vi "Test Lockin API - SM Sequencer.vi"() -> ()   [LabVIEW 2019]
uses:
  src/Instrument.Lockin/Instrument.Lockin.lvclass
  <vilib>/addons/_JKI Toolkits/Caraya/classes/Test Suite/Test Suite.lvclass
  src/Instrument.DAQ/Typedefs/Get State-enum.ctl
  <vilib>/addons/_JKI Toolkits/Caraya/classes/Assert/Assert Not Error.vi
  <vilib>/addons/_JKI Toolkits/Caraya/classes/Assert/Assert Equal Value_Variant.vi
  <vilib>/addons/_JKI Toolkits/Caraya/classes/Test Suite/Define Test Suite (Default).vi
  src/Instrument.DAQ/Typedefs/DAQ.Config.AO.Range--enum.ctl
  src/Instrument.DAQ/Instrument.DAQ.lvclass
  src/Instrument.DAQ/Typedefs/DAQ.Config.AI.Range--enum.ctl
  src/Instrument.DAQ/Typedefs/DAQ.Config.AI.Coupling--enum.ctl
  src/Instrument.DAQ/Typedefs/DAQ.Configuration--Cluster.ctl
  src/Instrument.DAQ/Typedefs/DAQ.Configuration--Cluster--Array.ctl
  <vilib>/addons/_JKI Toolkits/Caraya/classes/Assert/Assert.lvclass
panel:
  out "Current State":string
  in  "Tests":string
  in  "OK":bool
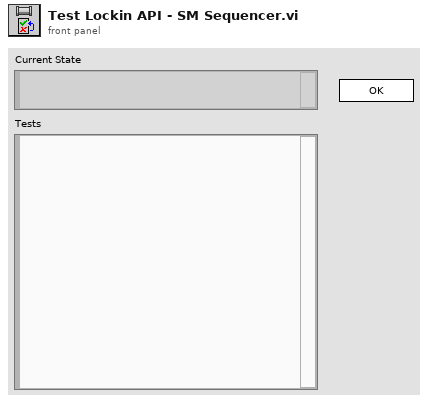
[diagram p1: front panel]
types:
  T1 = typedef "Instrument.DAQ.lvclass/DAQ.Configuration--Cluster--Array.ctl" = T2[]
  T2 = typedef "Instrument.DAQ.lvclass/DAQ.Configuration--Cluster.ctl" = cluster{"Device":string, "AO.Ch":string, "AO.Range":T3, "AI.Ch":string, "AI.Range":T4, "AI.Coupling":T5}
  T3 = typedef "Instrument.DAQ.lvclass/DAQ.Config.AO.Range--enum.ctl" = enum16{"±0.1", "±1.0", "±10.0"}
  T4 = typedef "Instrument.DAQ.lvclass/DAQ.Config.AI.Range--enum.ctl" = enum16{"±0.316", "±1.00", "±3.16", "±10.0", "±31.6", "±42.4"}
  T5 = typedef "Instrument.DAQ.lvclass/DAQ.Config.AI.Coupling--enum.ctl" = u16
  T6 = enum32{"Invalid", "Standard", "Closed", "Hidden", "Minimized", "Maximized"}
  T7 = enum32{"invalid app kind", "Development System", "Run Time System", "Student Edition", "Embedded LabVIEW", "Evaluation", "Custom"}
  T8 = typedef "Instrument.DAQ.lvclass/Get State-enum.ctl" = enum16{"idle", "created", "started", "stopped", "sweeping"}
  T9 = cluster{"Core":cluster{"Current VI Reference":refnum<vi>, "Close Panel on Exit?":bool}, "SelfRef":refnum<class "Instrument.Lockin.lvclass">, "Test Suite":refnum<class "Test Suite.lvclass">}
  T10 = cluster{"Current VI Reference":refnum<vi>, "Close Panel on Exit?":bool}
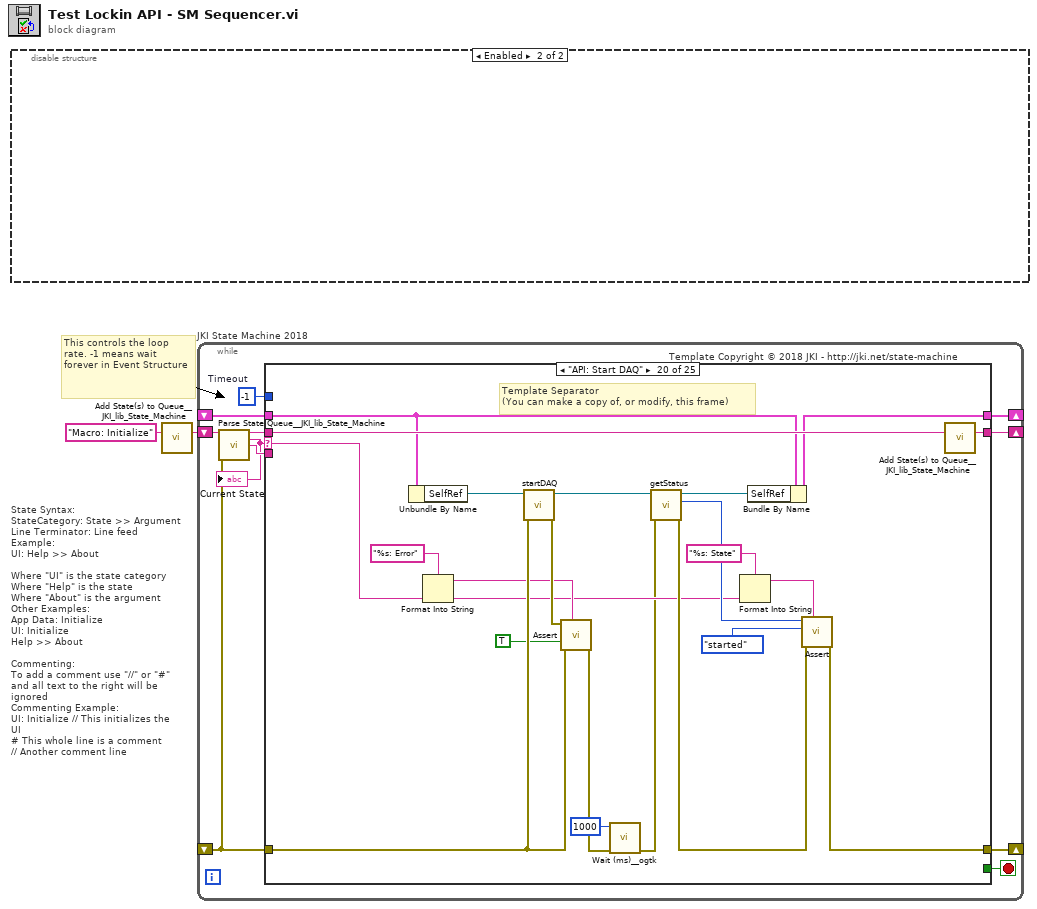
[diagram p0: block diagram]
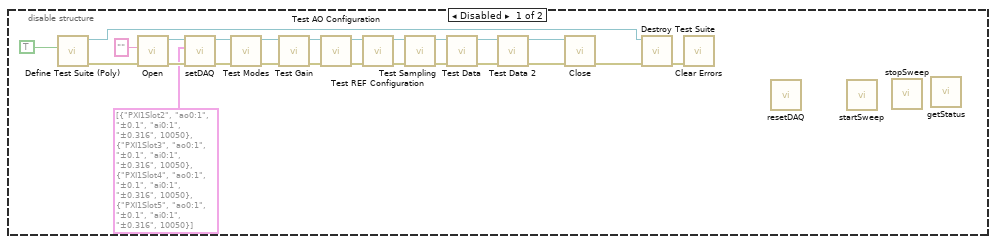
[diagram p2: hidden frame]
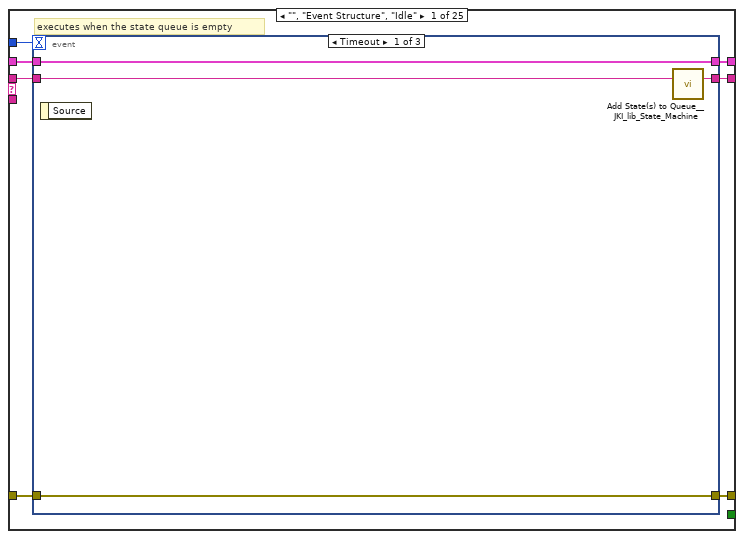
[diagram p3: hidden frame]
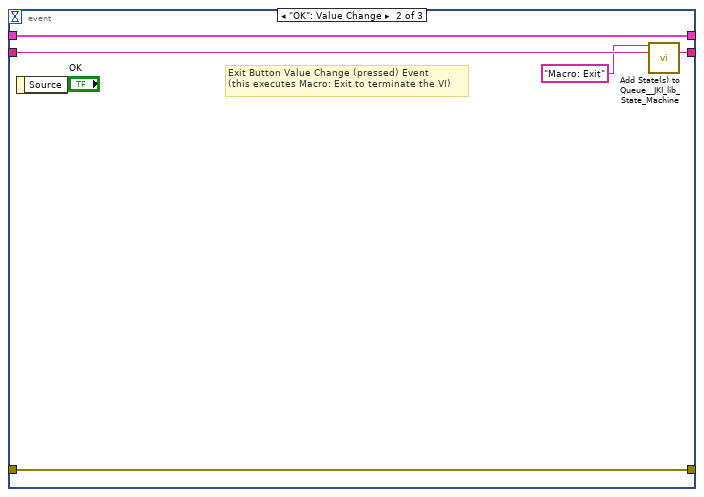
[diagram p4: hidden frame]
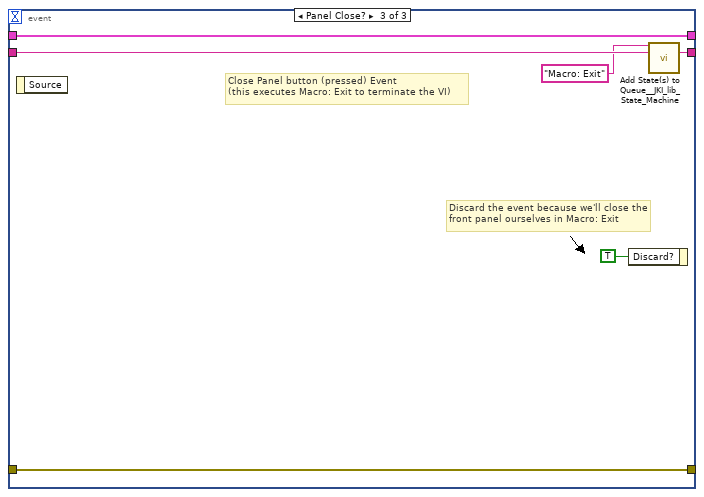
[diagram p5: hidden frame]
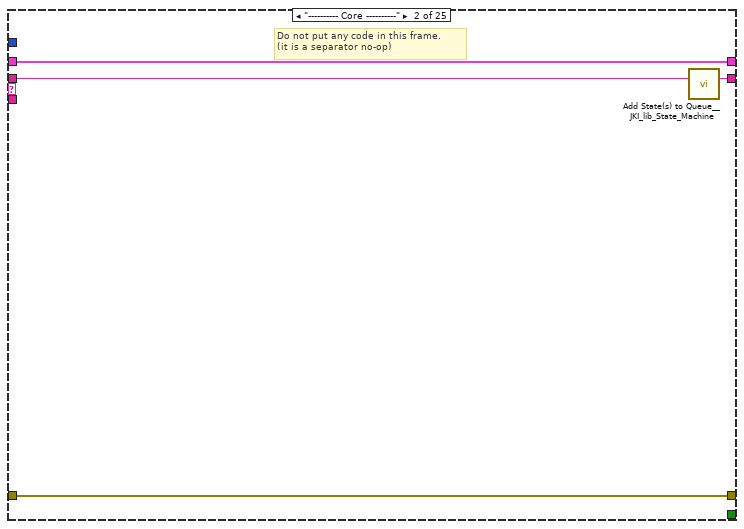
[diagram p6: hidden frame]
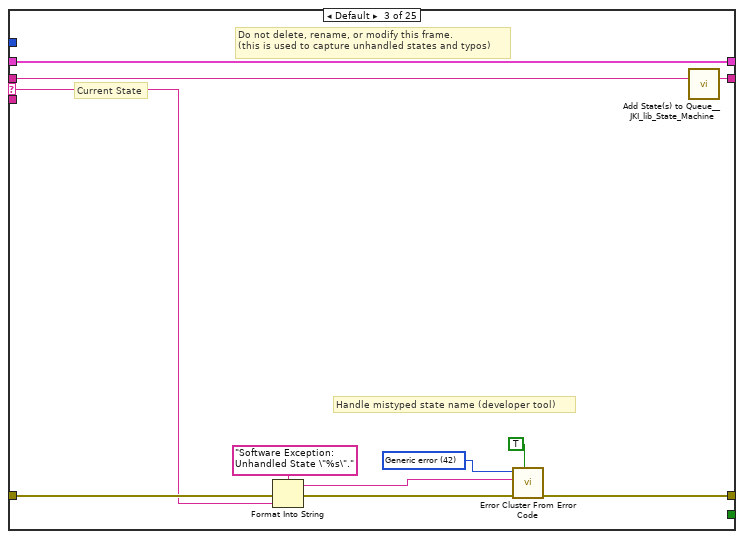
[diagram p7: hidden frame]
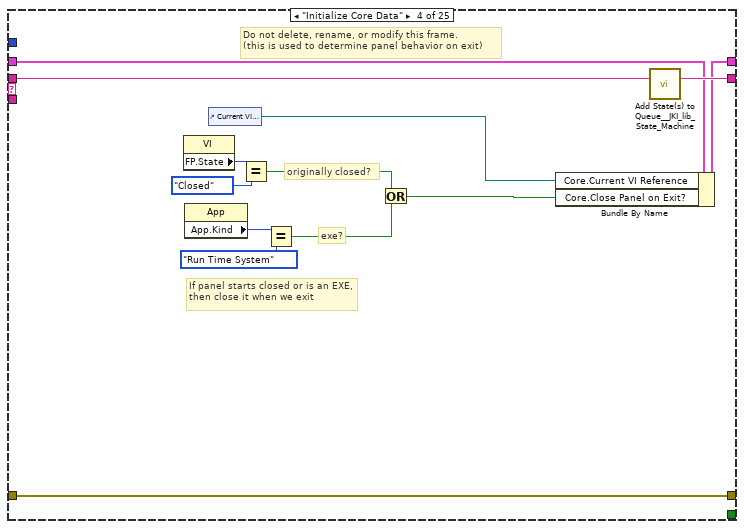
[diagram p8: hidden frame]
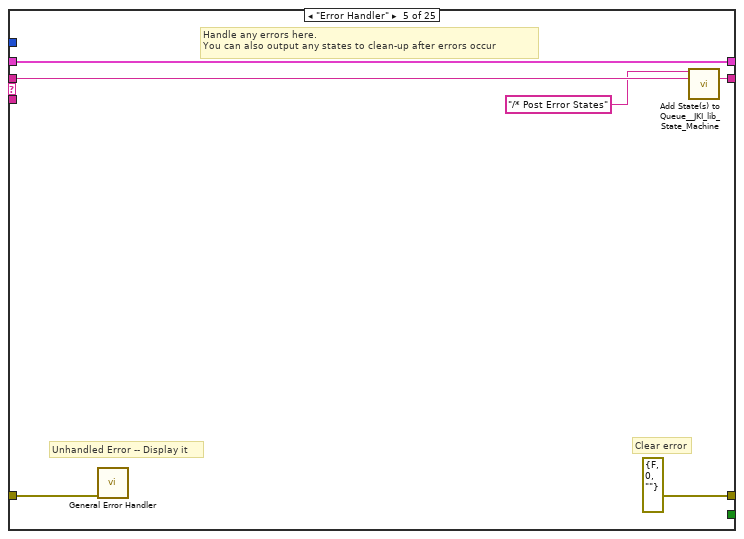
[diagram p9: hidden frame]
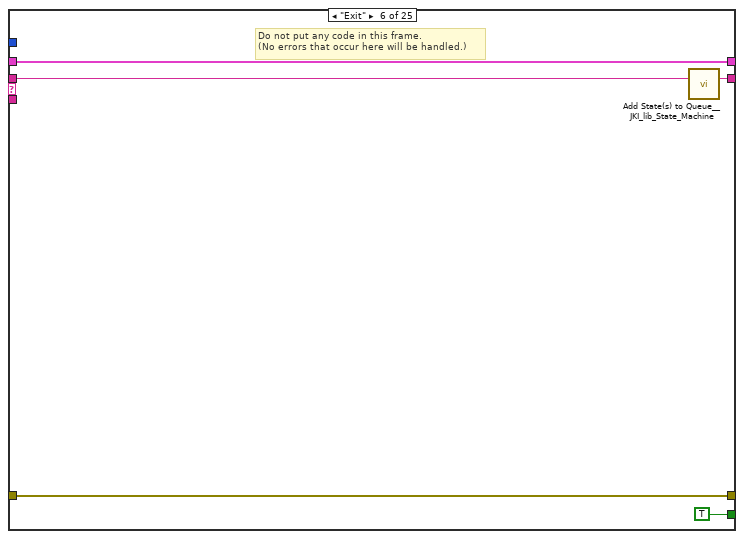
[diagram p10: hidden frame]
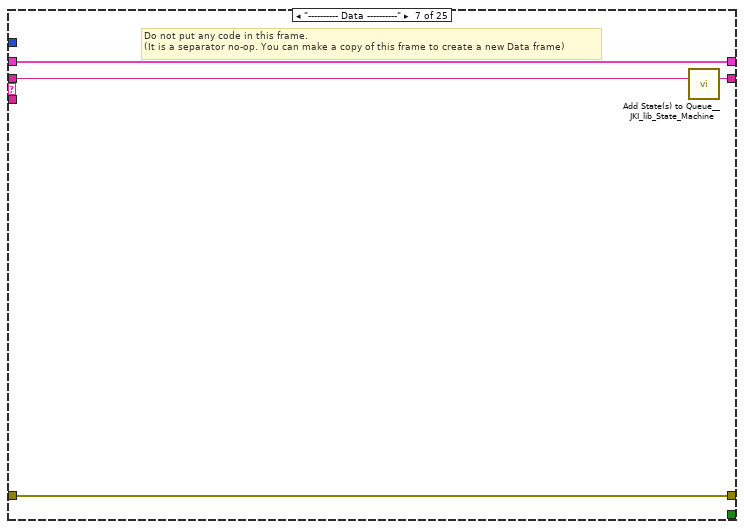
[diagram p11: hidden frame]
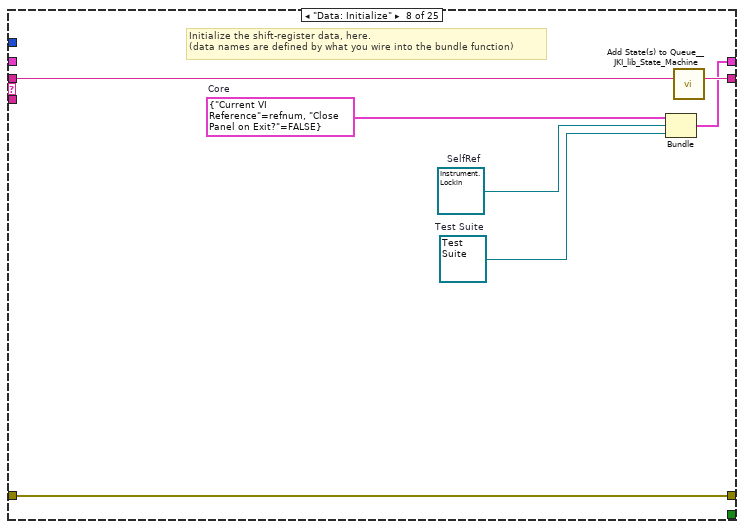
[diagram p12: hidden frame]
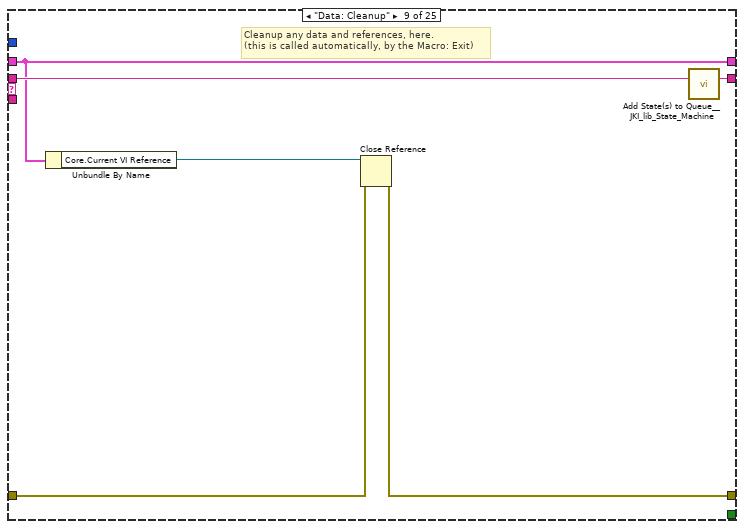
[diagram p13: hidden frame]
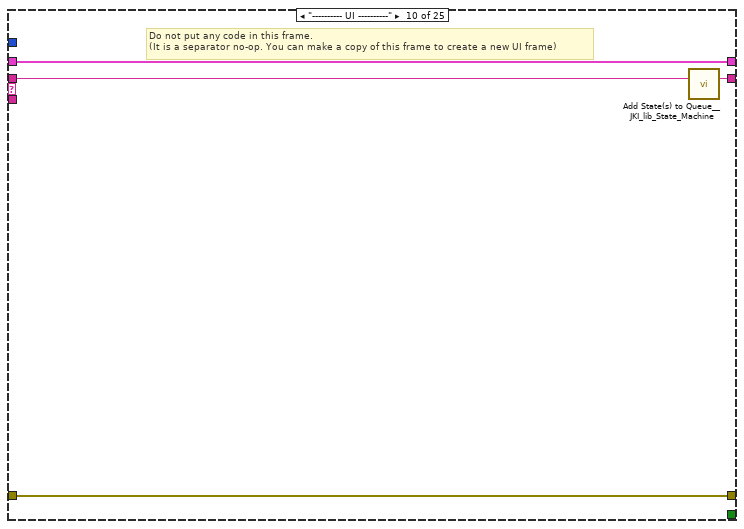
[diagram p14: hidden frame]
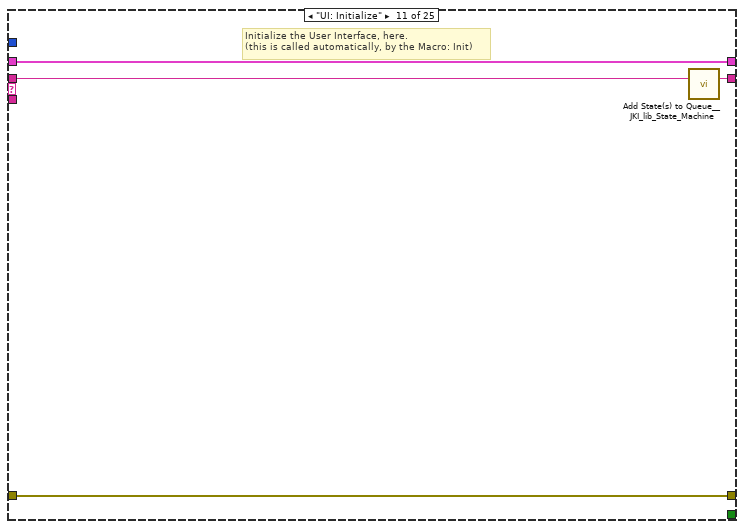
[diagram p15: hidden frame]
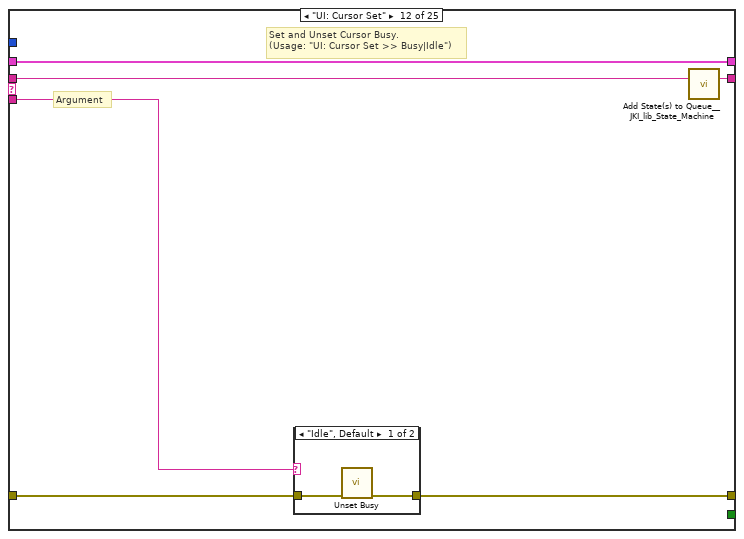
[diagram p16: hidden frame]
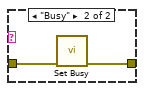
[diagram p17: hidden frame]
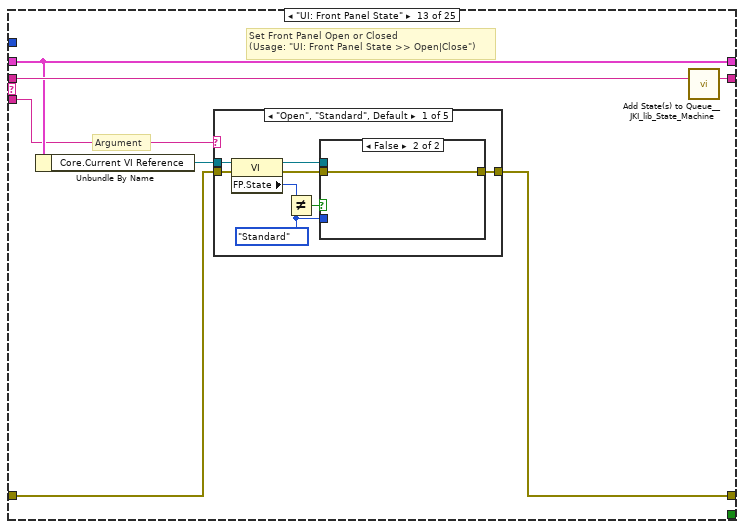
[diagram p18: hidden frame]
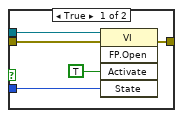
[diagram p19: hidden frame]
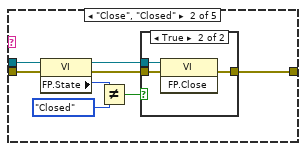
[diagram p20: hidden frame]
diagram:
  # "State Syntax:\nStateCategory: State >> Argument\nLine Terminator: Line feed\nExample:\nUI: Help >> About\n\nWhere \"UI\" is the state category\nWhere \"Help\" is the state\nWhere \"About\" is the argument\nOther Examples:\nApp Data: Initialize\nUI: Initialize\nHelp >> About\n\nCommenting:\nTo add a comment use \"//\" or \"#\" and all text to the right will be ignored\nCommenting Example:\nUI: Initialize // This initializes the UI\n# This whole line is a comment\n// Another comment line"
  # "This controls the loop rate. -1 means wait forever in Event Structure"
  n1 = disable-structure shown="Enabled" {
    frame Disabled {
      n2 = call-poly <vilib>:"Define Test Suite (Poly).vi"("Interactive"=TRUE) -> ("error out"=w14:errorcluster, "Test Suite"=w22:refnum<class "Test Suite.lvclass">)  [unwired: 9 in]
      n3 = call-dynamic "Open.vi"("error in (no error)"=w14, "address"="" ("Address")) -> ("error out"=w10:errorcluster, "Instrument.Lockin out"=w9:refnum<class "Instrument.Lockin.lvclass">)  [unwired: 8 in]
      n4 = call "setDAQ.vi"("error in (no error)"=w10, "setDAQ"=T1 [{"Device"="PXI1Slot2", "AO.Ch"="ao0:1", "AO.Range"=enum."±0.1", "AI.Ch"="ai0:1", "AI.Range"=enum."±0.316", "AI.Coupling"=10050}, {"Device"="PXI1Slot3", "AO.Ch"="ao0:1", "AO.Range"=enum."±0.1", "AI.Ch"="ai0:1", "AI.Range"=enum."±0.316", "AI.Coupling"=10050}, {"Device"="PXI1Slot4", "AO.Ch"="ao0:1", "AO.Range"=enum."±0.1", "AI.Ch"="ai0:1", "AI.Range"=enum."±0.316", "AI.Coupling"=10050}, {"Device"="PXI1Slot5", "AO.Ch"="ao0:1", "AO.Range"=enum."±0.1", "AI.Ch"="ai0:1", "AI.Range"=enum."±0.316", "AI.Coupling"=10050}], "Instrument.Lockin in"=w9) -> ("error out"=w7:errorcluster, "Instrument.Lockin out"=w8:refnum<class "Instrument.Lockin.lvclass">)  [unwired: 7 in]
      n5 = call "Test Modes.vi"("error in (no error)"=w7, "Instrument.Lockin in"=w8) -> ("error out"=w21:errorcluster, "Instrument.Lockin out"=w27:refnum<class "Instrument.Lockin.lvclass">)  [unwired: 8 in]
      n6 = call "Test Gain.vi"("error in (no error)"=w21, "Instrument.Lockin in"=w27) -> ("error out"=w20:errorcluster, "Instrument.Lockin out"=w26:refnum<class "Instrument.Lockin.lvclass">)  [unwired: 8 in]
      n7 = call "Test AO Configuration.vi"("error in (no error)"=w20, "Instrument.Lockin in"=w26) -> ("error out"=w19:errorcluster, "Instrument.Lockin out"=w25:refnum<class "Instrument.Lockin.lvclass">)  [unwired: 8 in]
      n8 = call "Test REF Configuration.vi"("error in (no error)"=w19, "Instrument.Lockin in"=w25) -> ("error out"=w18:errorcluster, "Instrument.Lockin out"=w24:refnum<class "Instrument.Lockin.lvclass">)  [unwired: 8 in]
      n9 = call "Test Sampling.vi"("error in (no error)"=w18, "Instrument.Lockin in"=w24) -> ("error out"=w17:errorcluster, "Instrument.Lockin out"=w23:refnum<class "Instrument.Lockin.lvclass">)  [unwired: 8 in]
      n10 = call "Test Data.vi"("error in (no error)"=w17, "Instrument.Lockin in"=w23) -> ("error out"=w12:errorcluster, "Instrument.Lockin out"=w11:refnum<class "Instrument.Lockin.lvclass">)  [unwired: 8 in]
      n11 = call "Test Data 2.vi"("error in (no error)"=w12, "Instrument.Lockin in"=w11) -> ("error out"=w4:errorcluster, "Instrument.Lockin out"=w5:refnum<class "Instrument.Lockin.lvclass">)  [unwired: 8 in]
      n12 = call-dynamic "Close.vi"("error in (no error)"=w4, "Instrument.Lockin in"=w5) -> ("error out"=w3:errorcluster)  [unwired: 8 in, 1 out]
      n13 = call-dynamic "Destroy Test Suite.vi"("error in (no error)"=w3, "Test Suite in"=w22) -> ("error out"=w15:errorcluster)  [unwired: 8 in, 1 out]
      n14 = call <vilib>:"Clear Errors.vi"("error in (no error)"=w15) -> ()  [unwired: 5 in, 2 out]
      n15 = call "resetDAQ.vi"() -> ()  [unwired: 10 in, 2 out]
      n16 = call "startSweep.vi"() -> ()  [unwired: 10 in, 2 out]
      n17 = call "stopSweep.vi"() -> ()  [unwired: 10 in, 2 out]
      n18 = call "getStatus.vi"() -> ()  [unwired: 9 in, 3 out]
    }
    frame Enabled {
    }
  }
  n19 = call <vilib>:"Add State(s) to Queue__JKI_lib_State_Machine.vi"("State(s) in (\"\")"="Macro: Initialize") -> ("States Out"=w2:string)  [unwired: 14 in]
  n20 = while "JKI State Machine 2018" {
    shift-right: [w32] -> _
    shift-left: _ -> [w29]
    shift-right: [w35] -> _
    shift-left: _ -> [w30]
    shift-right: [w34] -> _
    shift-left: w2 -> [w36]
    stop <- w33 stop-if-true
    w31 = -1  # Timeout
    # "Template Copyright © 2018 JKI - http://jki.net/state-machine"
    n21 = call <vilib>:"Parse State Queue__JKI_lib_State_Machine.vi"("State Queue"=w36, "Error In (no error)"=w30) -> ("Remaining States"=w38:string, "Current State"=w28:string, "Arguments"=w37:string)  [unwired: 11 in]
    "Current State" <- w28
    n22 = case shown="\"API: Start DAQ\"" w28 {
      selector: w28 -> [_ _ w65 _ _ _ _ _ _ _ _ _ _ _ _ _ _ w234 _ w259 w280 _ _ _ _]
      tunnel: w38 -> [w45 w64 w69 w88 w94 w99 w103 w110 w116 w120 w124 w130 w141 w210 w215 w223 w233 w244 w253 w275 w296 w304 w310 w318 w324]
      tunnel: w37 -> [_ _ _ _ _ _ _ _ _ _ _ w125 w135 _ _ _ _ _ _ _ _ _ _ _ _]
      tunnel: [w42 w62 w71 w85 errorcluster {"status"=FALSE, "code"=0, "source"=""} ("error out") w96 w101 w107 w112 w118 w121 w126 w138 w208 w213 w221 w231 w235 w251 w263 w284 w298 w308 w312 w321] -> w35
      tunnel: w30 -> [w41 w62 w70 w85 w90 w96 w101 w107 w113 w118 w121 w127 w139 w208 w213 w221 w231 w237 w250 w267 w288 w297 w308 w311 w320]
      tunnel: [w44 w63 w68 w87 w93 w98 w102 w109 w115 w119 w123 w129 w140 w209 w214 w222 w232 w243 w252 w274 w295 w303 w309 w317 w323] -> w34
      tunnel: [_ _ _ _ _ TRUE _ _ _ _ _ _ _ _ _ _ _ _ _ _ _ _ _ _ _] -> w33
      tunnel: [w40 w61 w67 w86 w91 w97 w100 w108 w111 w117 w122 w128 w137 w207 w212 w220 w230 w242 w247 w273 w294 w302 w306 w316 w319] -> w32
      tunnel: w31 -> [w39 _ _ _ _ _ _ _ _ _ _ _ _ _ _ _ _ _ _ _ _ _ _ _ _]
      tunnel: w29 -> [w43 w61 w67 w81 w91 w97 w100 _ w111 w117 w122 w128 w137 w207 w212 w220 w230 w241 w246 w272 w293 w301 w305 w315 w319]
      frame "", "Event Structure", "Idle" {
        # "executes when the state queue is empty"
        n23 = event shown="[0] Timeout" {
          selector: _ -> [_ _ _]
          dyn-events: _ -> [_ _ _]
          timeout: w39 -> [_ _ _]
          tunnel: w45 -> [w49 w54 w60]
          tunnel: [w48 w53 w59] -> w44
          tunnel: w43 -> [w46 w51 w57]
          tunnel: [w47 w52 w58] -> w42
          tunnel: w41 -> [w47 w52 w58]
          tunnel: [w46 w51 w57] -> w40
          event Timeout {
            n24 = event-data() -> ()  [unwired: 1 in, 1 out]
            n25 = call <vilib>:"Add State(s) to Queue__JKI_lib_State_Machine.vi"("State(s) in (\"\")"=w49) -> ("States Out"=w48:string)  [unwired: 14 in]
          }
          event "OK": Value Change {
            # "Exit Button Value Change (pressed) Event\n(this executes Macro: Exit to terminate the VI)"
            n26 = event-data() -> ()  [unwired: 1 in, 1 out]
            n27 = call <vilib>:"Add State(s) to Queue__JKI_lib_State_Machine.vi"("State(s) in Front (\"\")"="Macro: Exit", "State(s) in (\"\")"=w54) -> ("States Out"=w53:string)  [unwired: 13 in]
          }
          event Panel Close? {
            # "Discard the event because we'll close the front panel ourselves in Macro: Exit"
            # "Close Panel button (pressed) Event\n(this executes Macro: Exit to terminate the VI)"
            n28 = event-data() -> ()  [unwired: 1 in, 1 out]
            n29 = event-data("Discard?"=TRUE) -> ()  [unwired: 1 in, 1 out]
            n30 = call <vilib>:"Add State(s) to Queue__JKI_lib_State_Machine.vi"("State(s) in Front (\"\")"="Macro: Exit", "State(s) in (\"\")"=w60) -> ("States Out"=w59:string)  [unwired: 13 in]
          }
        }
      }
      frame "---------- Core ----------" {
        # "Do not put any code in this frame.\n(it is a separator no-op)"
        n31 = call <vilib>:"Add State(s) to Queue__JKI_lib_State_Machine.vi"("State(s) in (\"\")"=w64) -> ("States Out"=w63:string)  [unwired: 14 in]
      }
      frame Default {
        w74 = 42 items=["No error", "Argument error", "Memory is full", "Out of zone", "End of file", "File already open", "Generic file I/O error", "File not found", "File permission error", "Disk is full", "Duplicate path", "Too many files open", "System feature not enabled", "Resource file not found", "Cannot add resource", "Resource not found", "Image not found", "Image memory error", "Pen does not exist", "Config type invalid", "Config token not found", "Config parse error", "Config memory error", "Bad external code format", "Bad external code offset", "External code not present", "Null window", "Destroy window error", "Null menu", "Print aborted", "Bad print record", "Print driver error", "Windows error during printing", "Memory error during printing", "Print dialog error", "Generic print error", "Invalid device refnum", "Device not found", "Device parameter error", "Device unit error", "Cannot open device", "Device call aborted", "Generic error", "Cancelled by user", "Object ID too low", "Object ID too high", "Object not in heap", "Unknown heap", "Unknown object (invalid DefProc)", "Unknown object (DefProc not in table)", "Message out of range", "Invalid (null) method", "Unknown message", "Manager call not supported", "Bad address", "Network operation in progress", "Network operation timed out", "Connection is busy", "Network attribute not supported", "Network error", "Address in use", "System out of memory", "Connection aborted", "Connection refused", "Not connected", "Already connected", "Connection closed", "Initialization error (interapplication manager)", "Bad occurrence", "Wait on unbound occurrence handler", "Occurrence queue overflow", "Datalog type conflict", "Unused", "Unrecognized type (interapplication manager)", "Memory corrupt", "Failed to make temporary DLL", "Old CIN version", "Drag socket not found", "Failed to load drop-object", "Failed to register OLE object", "Failed to release OLE object", "Format specifier type mismatch", "Unknown format specifier", "Too few format specifiers", "Too many format specifiers", "Scan failed", "Newer CIN version", "Error converting to variant", "Runtime menu error", "Password tampered", "Variant attribute not found", "Incompatible variant data type", "Event data is not available", "Event Store is not present", "Occurrence is not found", "Event Queue is not created", "Event info is not available", "Refnum passed is NULL", "Error retrieving Class GUID", "Error retrieving CoClass GUID", "Error retrieving TypeLib GUID.", "Bad built application magic bytes.", "Specific driver is different from the specific driver associated with the Logical Name.", "There is no session opened to the class driver.", "Max Error", "MAX - Error with config objects", "MAX - Error loading configuration", "MAX - Group not supported"]
        # "Current State"
        # "Do not delete, rename, or modify this frame.\n(this is used to capture unhandled states and typos)"
        # "Handle mistyped state name (developer tool)"
        n32 = Format Into String(format string="Software Exception: Unhandled State \"%s\"." ("message"), error in=w70, w65) -> (resulting string=w73:string, error out=w72:errorcluster)  [unwired: 1 in]
        n33 = call <vilib>:"Error Cluster From Error Code.vi"("show call chain? (False)"=TRUE, "error in (no error)"=w72, "error message (\"\")"=w73, "error code (0)"=w74) -> ("error out"=w71:errorcluster)  [unwired: 5 in]
        n34 = call <vilib>:"Add State(s) to Queue__JKI_lib_State_Machine.vi"("State(s) in (\"\")"=w69) -> ("States Out"=w68:string)  [unwired: 14 in]
      }
      frame "Initialize Core Data" {
        # "Do not delete, rename, or modify this frame.\n(this is used to determine panel behavior on exit)"
        # "originally closed?"
        # "exe?"
        # "If panel starts closed or is an EXE, then close it when we exit"
        n35 = property class="VI"() -> ("FP.State"=w78:T6)  [unwired: 2 in, 2 out]
        n36 = property class="App"() -> ("App.Kind"=w84:T7)  [unwired: 2 in, 2 out]
        n37 = control-ref of="Current VI Reference"() -> (w79:refnum<vi>)
        n38 = Equal?(x=w78, y=T6."Closed" ("Front Panel Window:State")) -> (x = y?=w76:bool)
        n39 = Equal?(x=w84, y=T7."Run Time System" ("Application:Kind")) -> (x = y?=w82:bool)
        n40 = Or(x=w76, y=w82) -> (x .or. y?=w80:bool)
        n41 = Bundle By Name(cluster=w81, "Core.Current VI Reference"=w79, "Core.Close Panel on Exit?"=w80) -> (w86:T9)
        n42 = call <vilib>:"Add State(s) to Queue__JKI_lib_State_Machine.vi"("State(s) in (\"\")"=w88) -> ("States Out"=w87:string)  [unwired: 14 in]
      }
      frame "Error Handler" {
        # "Unhandled Error -- Display it"
        # "Handle any errors here.\nYou can also output any states to clean-up after errors occur"
        # "Clear error"
        n43 = call <vilib>:"General Error Handler.vi"("error in (no error)"=w90) -> ()  [unwired: 10 in, 5 out]
        n44 = call <vilib>:"Add State(s) to Queue__JKI_lib_State_Machine.vi"("State(s) in Front (\"\")"="/* Post Error States", "State(s) in (\"\")"=w94) -> ("States Out"=w93:string)  [unwired: 13 in]
      }
      frame "Exit" {
        # "Do not put any code in this frame.\n(No errors that occur here will be handled.)"
        n45 = call <vilib>:"Add State(s) to Queue__JKI_lib_State_Machine.vi"("State(s) in (\"\")"=w99) -> ("States Out"=w98:string)  [unwired: 14 in]
      }
      frame "---------- Data ----------" {
        # "Do not put any code in this frame.\n(It is a separator no-op. You can make a copy of this frame to create a new Data frame)"
        n46 = call <vilib>:"Add State(s) to Queue__JKI_lib_State_Machine.vi"("State(s) in (\"\")"=w103) -> ("States Out"=w102:string)  [unwired: 14 in]
      }
      frame "Data: Initialize" {
        w104 = refnum<class "Test Suite.lvclass"> refnum  # Test Suite
        w105 = refnum<class "Instrument.Lockin.lvclass"> refnum  # SelfRef
        w106 = T10 {"Current VI Reference"=refnum, "Close Panel on Exit?"=FALSE}  # Core
        # "Initialize the shift-register data, here.\n(data names are defined by what you wire into the bundle function)"
        n47 = Bundle("Core"=w106, "SelfRef"=w105, "Test Suite"=w104) -> (w108:T9)  [unwired: 1 in]
        n48 = call <vilib>:"Add State(s) to Queue__JKI_lib_State_Machine.vi"("State(s) in (\"\")"=w110) -> ("States Out"=w109:string)  [unwired: 14 in]
      }
      frame "Data: Cleanup" {
        # "Cleanup any data and references, here.\n(this is called automatically, by the Macro: Exit)"
        n49 = Unbundle By Name(w111) -> ("Core.Current VI Reference"=w114:refnum<vi>)
        n50 = Close Reference(reference=w114, error in (no error)=w113) -> (error out=w112:errorcluster)
        n51 = call <vilib>:"Add State(s) to Queue__JKI_lib_State_Machine.vi"("State(s) in (\"\")"=w116) -> ("States Out"=w115:string)  [unwired: 14 in]
      }
      frame "---------- UI ----------" {
        # "Do not put any code in this frame.\n(It is a separator no-op. You can make a copy of this frame to create a new UI frame)"
        n52 = call <vilib>:"Add State(s) to Queue__JKI_lib_State_Machine.vi"("State(s) in (\"\")"=w120) -> ("States Out"=w119:string)  [unwired: 14 in]
      }
      frame "UI: Initialize" {
        # "Initialize the User Interface, here.\n(this is called automatically, by the Macro: Init)"
        n53 = call <vilib>:"Add State(s) to Queue__JKI_lib_State_Machine.vi"("State(s) in (\"\")"=w124) -> ("States Out"=w123:string)  [unwired: 14 in]
      }
      frame "UI: Cursor Set" {
        # "Argument"
        # "Set and Unset Cursor Busy.\n(Usage: \"UI: Cursor Set >> Busy|Idle\")"
        n54 = case shown="\"Idle\", Default" w125 {
          tunnel: w127 -> [w132 w134]
          tunnel: [w131 w133] -> w126
          frame "Idle", Default {
            n55 = call <vilib>:"Unset Busy.vi"("error in (no error)"=w132) -> ("error out"=w131:errorcluster)  [unwired: 10 in]
          }
          frame "Busy" {
            n56 = call <vilib>:"Set Busy.vi"("error in (no error)"=w134) -> ("error out"=w133:errorcluster)  [unwired: 9 in, 1 out]
          }
        }
        n57 = call <vilib>:"Add State(s) to Queue__JKI_lib_State_Machine.vi"("State(s) in (\"\")"=w130) -> ("States Out"=w129:string)  [unwired: 14 in]
      }
      frame "UI: Front Panel State" {
        # "Argument"
        # "Set Front Panel Open or Closed\n(Usage: \"UI: Front Panel State >> Open|Close\")"
        n58 = Unbundle By Name(w137) -> ("Core.Current VI Reference"=w136:refnum<vi>)
        n59 = case shown="\"Open\", \"Standard\", Default" w135 {
          tunnel: w139 -> [w147 w162 w173 w186 w199]
          tunnel: [w149 w163 w175 w188 w201] -> w138
          tunnel: w136 -> [w148 w160 w174 w187 w200]
          frame "Open", "Standard", Default {
            w142 = T6."Standard" ("State")
            n60 = property class="VI"(reference=w148, error in=w147) -> (reference out=w145:refnum<vi>, error out=w146:errorcluster, "FP.State"=w144:T6)
            n61 = Not Equal?(x=w144, y=w142) -> (x != y?=w143:bool)
            n62 = case shown="False" w143 {
              tunnel: [w153 w155] -> w149
              tunnel: w146 -> [w152 w155]
              tunnel: w145 -> [w151 _]
              tunnel: w142 -> [w150 _]
              frame True {
                n63 = invoke class="VI" method="FP.Open"(reference=w151, error in=w152, "Activate"=TRUE, "State"=w150) -> (error out=w153:errorcluster)  [unwired: 1 in, 4 out]
              }
              frame False {
              }
            }
          }
          frame "Close", "Closed" {
            n64 = property class="VI"(reference=w160, error in=w162) -> (reference out=w159:refnum<vi>, error out=w161:errorcluster, "FP.State"=w157:T6)
            n65 = Not Equal?(x=w157, y=T6."Closed" ("Front Panel Window:State")) -> (x != y?=w156:bool)
            n66 = case shown="True" w156 {
              tunnel: [w164 w167] -> w163
              tunnel: w161 -> [w164 w166]
              tunnel: w159 -> [_ w165]
              frame False {
              }
              frame True {
                n67 = invoke class="VI" method="FP.Close"(reference=w165, error in=w166) -> (error out=w167:errorcluster)  [unwired: 1 in, 2 out]
              }
            }
          }
          frame "Hidden", "Hide" {
            w168 = T6."Hidden" ("State")
            n68 = property class="VI"(reference=w174, error in=w173) -> (reference out=w171:refnum<vi>, error out=w172:errorcluster, "FP.State"=w170:T6)
            n69 = Not Equal?(x=w170, y=w168) -> (x != y?=w169:bool)
            n70 = case shown="True" w169 {
              tunnel: [w179 w180] -> w175
              tunnel: w172 -> [w178 w180]
              tunnel: w171 -> [w177 _]
              tunnel: w168 -> [w176 _]
              frame True {
                n71 = invoke class="VI" method="FP.Open"(reference=w177, error in=w178, "State"=w176) -> (error out=w179:errorcluster)  [unwired: 2 in, 4 out]
              }
              frame False {
              }
            }
          }
          frame "Minimize", "Minimized" {
            w181 = T6."Minimized" ("State")
            n72 = property class="VI"(reference=w187, error in=w186) -> (reference out=w184:refnum<vi>, error out=w185:errorcluster, "FP.State"=w183:T6)
            n73 = Not Equal?(x=w183, y=w181) -> (x != y?=w182:bool)
            n74 = case shown="False" w182 {
              tunnel: [w192 w193] -> w188
              tunnel: w185 -> [w191 w193]
              tunnel: w184 -> [w190 _]
              tunnel: w181 -> [w189 _]
              frame True {
                n75 = invoke class="VI" method="FP.Open"(reference=w190, error in=w191, "State"=w189) -> (error out=w192:errorcluster)  [unwired: 2 in, 4 out]
              }
              frame False {
              }
            }
          }
          frame "Maximize", "Maximized" {
            w194 = T6."Maximized" ("State")
            n76 = property class="VI"(reference=w200, error in=w199) -> (reference out=w197:refnum<vi>, error out=w198:errorcluster, "FP.State"=w196:T6)
            n77 = Not Equal?(x=w196, y=w194) -> (x != y?=w195:bool)
            n78 = case shown="True" w195 {
              tunnel: [w205 w206] -> w201
              tunnel: w198 -> [w204 w206]
              tunnel: w197 -> [w203 _]
              tunnel: w194 -> [w202 _]
              frame True {
                n79 = invoke class="VI" method="FP.Open"(reference=w203, error in=w204, "State"=w202) -> (error out=w205:errorcluster)  [unwired: 2 in, 4 out]
              }
              frame False {
              }
            }
          }
        }
        n80 = call <vilib>:"Add State(s) to Queue__JKI_lib_State_Machine.vi"("State(s) in (\"\")"=w141) -> ("States Out"=w140:string)  [unwired: 14 in]
      }
      frame "---------- Macro ----------" {
        # "Do not put any code in this frame.\n(It is a separator no-op. You can make a copy of this frame to create a new Macro frame)"
        n81 = call <vilib>:"Add State(s) to Queue__JKI_lib_State_Machine.vi"("State(s) in (\"\")"=w210) -> ("States Out"=w209:string)  [unwired: 14 in]
      }
      frame "Macro: Initialize" {
        w211 = "Data: Initialize\nInitialize Core Data\nUI: Initialize\nUI: Front Panel State >> Open\nMacro: Tests"  # Data: Initialize Initialize Core Data UI: Initialize UI: Front Panel State >> Open Macro: Tests
        # "Initialization Macro\n(This is called once, when the VI starts)"
        n82 = call <vilib>:"Add State(s) to Queue__JKI_lib_State_Machine.vi"("State(s) in Front (\"\")"=w211, "State(s) in (\"\")"=w215) -> ("States Out"=w214:string)  [unwired: 13 in]
      }
      frame "Macro: Tests" {
        # "API: Open\nAPI: Start DAQ\nAPI: Stop DAQ\nAPI: Close"
        # "Do not put any code in this frame.\n(It is a separator no-op. You can make a copy of this frame to create a new Macro frame)"
        n83 = call <vilib>:"Add State(s) to Queue__jki_lib_state_machine.vi"("State(s) in Front (\"\")"="Test: Define" ("State(s) at Back (\"\")"), "State(s) in (\"\")"="Tests", "State(s) at Back (\"\")"="Test: Destroy\nMacro: Exit" ("State(s) at Back (\"\")")) -> ("States Out"=w216:string)  [unwired: 12 in]
        n84 = call <vilib>:"Add State(s) to Queue__JKI_lib_State_Machine.vi"("State(s) in Front (\"\")"=w216, "State(s) in (\"\")"=w223) -> ("States Out"=w222:string)  [unwired: 13 in]
      }
      frame "Macro: Exit" {
        # "Exit Macro\n(This is called once, when the VI exits)"
        n85 = Unbundle By Name(w230) -> ("Core.Close Panel on Exit?"=w229:bool)
        n86 = Select(t="UI: Front Panel State >> Close", s=w229, f="") -> (s? t:f=w226:string)
        n87 = call <vilib>:"Add State(s) to Queue__JKI_lib_State_Machine.vi"("State(s) in (\"\")"=w226, "State(s) at Back (\"\")"="Data: Cleanup\nExit") -> ("States Out"=w224:string)  [unwired: 13 in]
        n88 = call <vilib>:"Add State(s) to Queue__JKI_lib_State_Machine.vi"("State(s) in Front (\"\")"=w224, "State(s) in (\"\")"=w233) -> ("States Out"=w232:string)  [unwired: 13 in]
      }
      frame "---------- API ----------" {
        # "Template Separator\n(You can make a copy of, or modify, this frame)"
        n89 = Unbundle By Name(w241) -> ("SelfRef"=w240:refnum<class "Instrument.Lockin.lvclass">)
        n90 = call-dynamic "Open.vi"("error in (no error)"=w237, "address"="" ("Address"), "Instrument.Lockin in"=w240) -> ("error out"=w236:errorcluster, "Instrument.Lockin out"=w238:refnum<class "Instrument.Lockin.lvclass">)  [unwired: 7 in]
        n91 = call-poly <vilib>:"Assert.vi"("Label"=w234, "error in (no error)"=w237, "Not Error?"=w236) -> ("error out"=w235:errorcluster)  [unwired: 8 in]
        n92 = Bundle By Name(cluster=w241, "SelfRef"=w238) -> (w242:T9)
        n93 = call <vilib>:"Add State(s) to Queue__JKI_lib_State_Machine.vi"("State(s) in (\"\")"=w244) -> ("States Out"=w243:string)  [unwired: 14 in]
      }
      frame "API: Open" {
        # "Your code here.\n(You can make a copy of, or modify, this frame)"
        n94 = Unbundle By Name(w246) -> ("SelfRef"=w245:refnum<class "Instrument.Lockin.lvclass">)
        n95 = call-dynamic "Open.vi"("error in (no error)"=w250, "address"="" ("Address"), "Instrument.Lockin in"=w245) -> ("error out"=w251:errorcluster, "Instrument.Lockin out"=w249:refnum<class "Instrument.Lockin.lvclass">)  [unwired: 7 in]
        n96 = Bundle By Name(cluster=w246, "SelfRef"=w249) -> (w247:T9)
        n97 = call <vilib>:"Add State(s) to Queue__JKI_lib_State_Machine.vi"("State(s) in (\"\")"=w253) -> ("States Out"=w252:string)  [unwired: 14 in]
      }
      frame "API: Start DAQ" {
        # "Template Separator\n(You can make a copy of, or modify, this frame)"
        n98 = Unbundle By Name(w272) -> ("SelfRef"=w271:refnum<class "Instrument.Lockin.lvclass">)
        n99 = Format Into String(format string="%s: Error", w259) -> (resulting string=w261:string)  [unwired: 2 in, 1 out]
        n100 = call "startDAQ.vi"("error in (no error)"=w267, "Instrument.Lockin in"=w271) -> ("error out"=w270:errorcluster, "Instrument.Lockin out"=w269:refnum<class "Instrument.Lockin.lvclass">)  [unwired: 8 in]
        n101 = call-poly <vilib>:"Assert.vi"("Label"=w261, "error in (no error)"=w267, "Register with caller test (F)"=TRUE, "Not Error?"=w270) -> ("error out"=w256:errorcluster)  [unwired: 7 in]
        n102 = call <userlib>:"Wait (ms)__ogtk.vi"("error in (no error)"=w256, "milliseconds to wait"=u32 1000) -> ("error out"=w255:errorcluster)  [unwired: 8 in, 1 out]
        n103 = call "getStatus.vi"("error in (no error)"=w255, "Instrument.Lockin"=w269) -> ("error out"=w264:errorcluster, "Status"=w265:T8, "Instrument.Lockin"=w268:refnum<class "Instrument.Lockin.lvclass">)  [unwired: 7 in]
        n104 = Format Into String(format string="%s: State", w259) -> (resulting string=w258:string)  [unwired: 2 in, 1 out]
        n105 = Bundle By Name(cluster=w272, "SelfRef"=w268) -> (w273:T9)
        n106 = call-poly <vilib>:"Assert.vi"("Label"=w258, "error in (no error)"=w264, "Y"=Get_State-enum."started" ("Status"), "X"=w265) -> ("error out"=w263:errorcluster)  [unwired: 7 in]
        n107 = call <vilib>:"Add State(s) to Queue__JKI_lib_State_Machine.vi"("State(s) in (\"\")"=w275) -> ("States Out"=w274:string)  [unwired: 14 in]
      }
      frame "API: Stop DAQ" {
        # "Template Separator\n(You can make a copy of, or modify, this frame)"
        n108 = Unbundle By Name(w293) -> ("SelfRef"=w292:refnum<class "Instrument.Lockin.lvclass">)
        n109 = Format Into String(format string="%s: Error", w280) -> (resulting string=w282:string)  [unwired: 2 in, 1 out]
        n110 = call "stopDAQ.vi"("error in (no error)"=w288, "Instrument.Lockin in"=w292) -> ("error out"=w291:errorcluster, "Instrument.Lockin out"=w290:refnum<class "Instrument.Lockin.lvclass">)  [unwired: 8 in]
        n111 = call-poly <vilib>:"Assert.vi"("Label"=w282, "error in (no error)"=w288, "Not Error?"=w291) -> ("error out"=w276:errorcluster)  [unwired: 8 in]
        n112 = call <userlib>:"Wait (ms)__ogtk.vi"("error in (no error)"=w276, "milliseconds to wait"=u32 1000) -> ("error out"=w278:errorcluster)  [unwired: 8 in, 1 out]
        n113 = call "getStatus.vi"("error in (no error)"=w278, "Instrument.Lockin"=w290) -> ("error out"=w285:errorcluster, "Status"=w286:T8, "Instrument.Lockin"=w289:refnum<class "Instrument.Lockin.lvclass">)  [unwired: 7 in]
        n114 = Format Into String(format string="%s: State", w280) -> (resulting string=w279:string)  [unwired: 2 in, 1 out]
        n115 = Bundle By Name(cluster=w293, "SelfRef"=w289) -> (w294:T9)
        n116 = call-poly <vilib>:"Assert.vi"("Label"=w279, "error in (no error)"=w285, "Y"=Get_State-enum."idle" ("Status"), "X"=w286) -> ("error out"=w284:errorcluster)  [unwired: 7 in]
        n117 = call <vilib>:"Add State(s) to Queue__JKI_lib_State_Machine.vi"("State(s) in (\"\")"=w296) -> ("States Out"=w295:string)  [unwired: 14 in]
      }
      frame "API: Close" {
        # "Template Separator\n(You can make a copy of, or modify, this frame)"
        n118 = Unbundle By Name(w301) -> ("SelfRef"=w300:refnum<class "Instrument.Lockin.lvclass">)
        n119 = call-dynamic "Close.vi"("error in (no error)"=w297, "Instrument.Lockin in"=w300) -> ("error out"=w298:errorcluster, "Instrument.Lockin out"=w299:refnum<class "Instrument.Lockin.lvclass">)  [unwired: 8 in]
        n120 = Bundle By Name(cluster=w301, "SelfRef"=w299) -> (w302:T9)
        n121 = call <vilib>:"Add State(s) to Queue__JKI_lib_State_Machine.vi"("State(s) in (\"\")"=w304) -> ("States Out"=w303:string)  [unwired: 14 in]
      }
      frame "---------- Test ----------" {
        # "Template Separator\n(You can make a copy of, or modify, this frame)"
        n122 = Unbundle By Name(w305) -> ("SelfRef"=w307:refnum<class "Instrument.Lockin.lvclass">)
        n123 = Bundle By Name(cluster=w305, "SelfRef"=w307) -> (w306:T9)
        n124 = call <vilib>:"Add State(s) to Queue__JKI_lib_State_Machine.vi"("State(s) in (\"\")"=w310) -> ("States Out"=w309:string)  [unwired: 14 in]
      }
      frame "Test: Define" {
        # "Template Separator\n(You can make a copy of, or modify, this frame)"
        n125 = call-poly <vilib>:"Define Test Suite (Poly).vi"("error in (no error)"=w311, "Interactive"=TRUE) -> ("error out"=w312:errorcluster, "Test Suite"=w313:refnum<class "Test Suite.lvclass">)  [unwired: 8 in]
        n126 = Bundle By Name(cluster=w315, "Test Suite"=w313) -> (w316:T9)
        n127 = call <vilib>:"Add State(s) to Queue__JKI_lib_State_Machine.vi"("State(s) in (\"\")"=w318) -> ("States Out"=w317:string)  [unwired: 14 in]
      }
      frame "Test: Destroy" {
        # "Template Separator\n(You can make a copy of, or modify, this frame)"
        n128 = Unbundle By Name(w319) -> ("Test Suite"=w322:refnum<class "Test Suite.lvclass">)
        n129 = call-dynamic "Destroy Test Suite.vi"("error in (no error)"=w320, "Test Suite in"=w322) -> ("error out"=w321:errorcluster)  [unwired: 8 in, 1 out]
        n130 = call <vilib>:"Add State(s) to Queue__JKI_lib_State_Machine.vi"("State(s) in (\"\")"=w324) -> ("States Out"=w323:string)  [unwired: 14 in]
      }
    }
  }
